vi "_FPGA Set Parameters.vi"(4 "HV Only (F)":bool, 5 "Source Standby (F)":bool, 6 "ExhaustGas (on)":bool=TRUE, 7 "CurGas (on)":bool=TRUE, 8 "error in":errorcluster, 9 "Set Zero (on)":bool=TRUE, 10 "HSID Temp (on)":bool=TRUE) -> (0 "error out":errorcluster)   [LabVIEW 2012]
uses:
  Type/_RT Active Ch.ctl
  Type/_RT Parameter.ctl
  Type/_RT Expt.ctl
  Type/_Run Mode.ctl
  Type/_RT Mass Range.ctl
  Type/_RT Res Type.ctl
  Type/_FPGA Indicator.ctl
  _RT Global.vi
  <vilib>/Utility/error.llb/Error Cluster From Error Code.vi
  <vilib>/rvi/errors/niLvFpgaAdjustHostInterfaceError.vi
  <vilib>/rvi/interface/nirviReadWriteControl/nirviReadWriteControl.xnode
  FPGA Bitfiles/FPGA9606.lvbitx
  NiFpgaLv.dll
panel:
  out "Array":T1[](array[typedef])
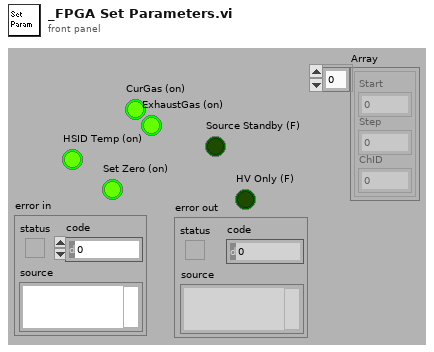
[diagram p1: front panel]
types:
  T1 = typedef "_RT Active Ch.ctl" = cluster{"Start":i32, "Step":i32, "ChID":i32}
  T2 = typedef "_RT Expt.ctl" = cluster{"StartT(mS)":i32, "#Cycles":i32, "Scan Type":T3, "PauseT(uS)":i32, "Polarity":u8, "DelayT(mS)":i32, "Active Ch":T1[], "Mass Range":T4[]}
  T3 = typedef "_Run Mode.ctl" = enum16{"MRM (Q1/Q2)", "Q1 Scan", "Q1 SRM", "Q2 Scan", "Q2 SRM", "Product Scan", "Precursor Scan", "Neutral Loss", "Neutral Gain"}
  T4 = typedef "_RT Mass Range.ctl" = cluster{"Steps":i32, "Dwell(uS)":i32, "Resolution Type":T5, "Ramping Ch":T1[]}
  T5 = typedef "_RT Res Type.ctl" = u16
  T6 = typedef "_RT Parameter.ctl" = cluster{"RunMode":i32, "Initial Ch":T1[], "Sync":u8, "Expt":T2[], "EqTime(mS)":i32}
  T7 = typedef "_RT Instrument 2.ctl" = cluster{"Table":T8[], "Instrument":string[]}
  T8 = typedef "_RT Configuration 2.ctl" = cluster{"Name":string, "Ch#":u8, "Min":dbl, "Max":dbl, "Def+":dbl, "Def-":dbl, "Offset":dbl, "Slope":dbl, "Type":u8, "Description":string, "SettleT":dbl}
  T9 = typedef "Semaphore RefNum" = refnum<k1>
  T10 = typedef "_FPGA Indicator.ctl" = enum16{"Done", "Ready", "Count Available", "SendSerial", "LED State"}
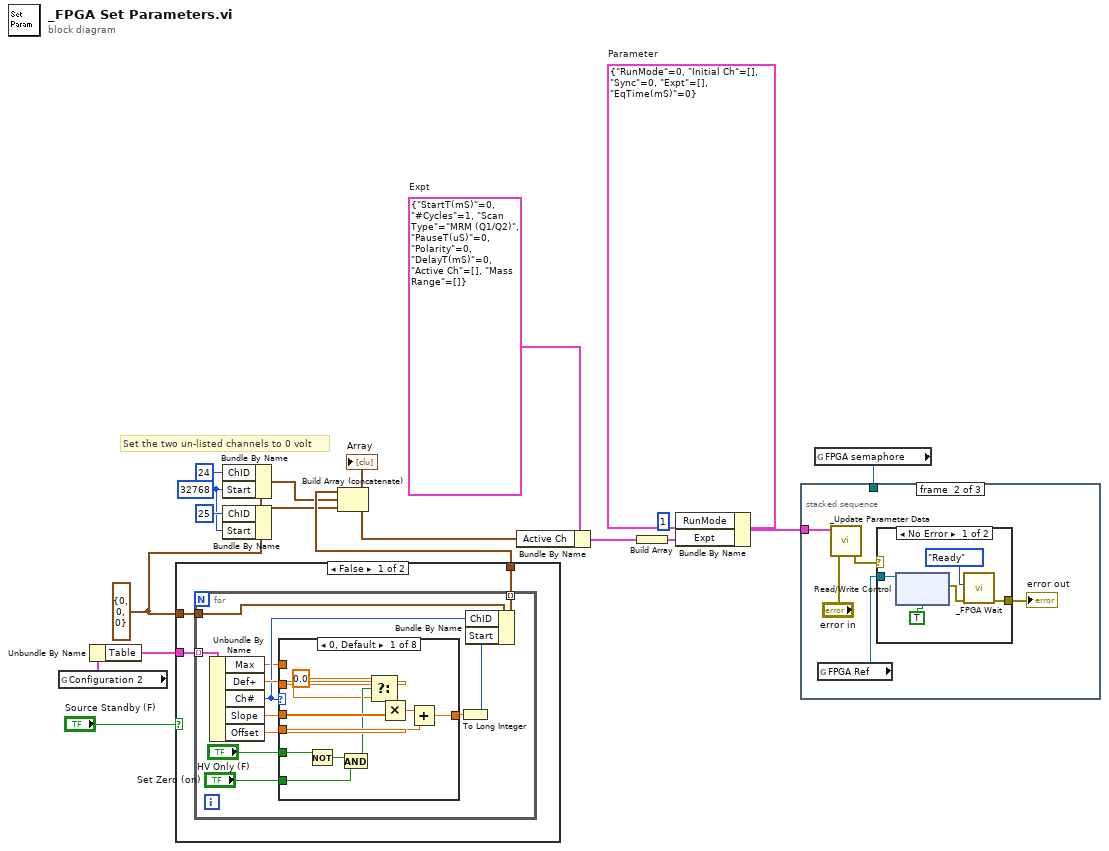
[diagram p0: block diagram]
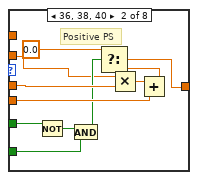
[diagram p2: hidden frame]
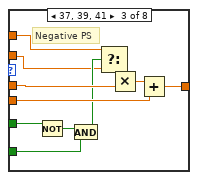
[diagram p3: hidden frame]
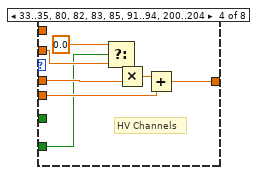
[diagram p4: hidden frame]
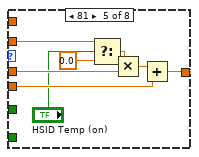
[diagram p5: hidden frame]
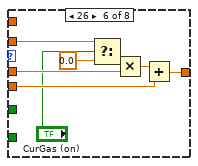
[diagram p6: hidden frame]
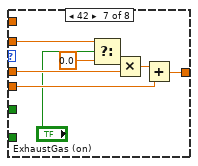
[diagram p7: hidden frame]
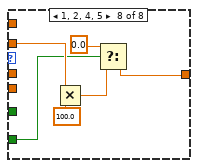
[diagram p8: hidden frame]
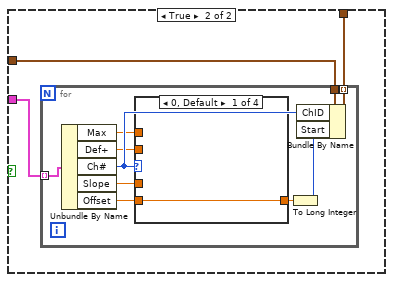
[diagram p9: hidden frame]
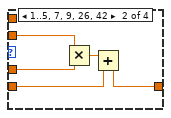
[diagram p10: hidden frame]
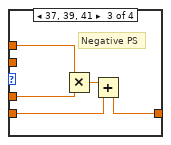
[diagram p11: hidden frame]
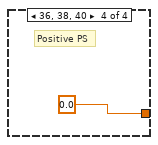
[diagram p12: hidden frame]
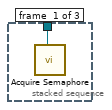
[diagram p13: hidden frame]
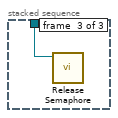
[diagram p15: hidden frame]
diagram:
  w5 = 32768 ("Start")
  w8 = T1 {"Start"=0, "Step"=0, "ChID"=0} ("Active Channel")
  w16 = T2 {"StartT(mS)"=0, "#Cycles"=1, "Scan Type"=enum."MRM (Q1/Q2)", "PauseT(uS)"=0, "Polarity"=0, "DelayT(mS)"=0, "Active Ch"=[], "Mass Range"=[]}  # Expt
  w15 = T6 {"RunMode"=0, "Initial Ch"=[], "Sync"=0, "Expt"=[], "EqTime(mS)"=0}  # Parameter
  # "Set the two un-listed channels to 0 volt"
  n1 = global read "_RT Global.vi" "Configuration 2"() -> (w11:T7)
  n2 = Unbundle By Name(w11) -> ("Table"=w17:T8[])
  n3 = case shown="False" "Source Standby (F)" {
    tunnel: [w21 w105] -> w4
    tunnel: w17 -> [w20 w106]
    tunnel: w8 -> [w19 w107]
    frame False {
      n4 = for {
        tunnel: w20 -> [w33] mode=indexing
        tunnel: [w32] -> w21 mode=indexing
        tunnel: w19 -> [w24]
        n5 = Unbundle By Name(w33) -> ("Max"=w22:dbl, "Def+"=w31:dbl, "Ch#"=w26:u8, "Slope"=w30:dbl, "Offset"=w29:dbl)
        n6 = case shown="0, Default" w26 {
          tunnel: w31 -> [w36 w47 w57 w70 w77 w84 w92 w103]
          tunnel: w30 -> [w44 w55 w66 w74 w82 w90 w98 _]
          tunnel: w29 -> [w43 w54 w65 w73 w81 w89 w97 _]
          tunnel: [w34 w45 w62 w68 w76 w85 w93 w99] -> w28
          tunnel: "Set Zero (on)" -> [w39 w50 w60 w67 _ _ _ w102]
          tunnel: "HV Only (F)" -> [w37 w48 w58 _ _ _ _ _]
          tunnel: w22 -> [_ _ w56 _ _ _ _ _]
          frame 0, Default {
            n7 = Not(x=w37) -> (.not. x?=w40:bool)
            n8 = And(x=w40, y=w39) -> (x .and. y?=w38:bool)
            n9 = Select(t=0.0 ("f"), s=w38, f=w36) -> (s? t:f=w35:dbl)
            n10 = Multiply(x=w35, y=w44) -> (x*y=w42:dbl)
            n11 = Add(x=w42, y=w43) -> (x+y=w34:dbl)
          }
          frame 36, 38, 40 {
            # "Positive PS"
            n12 = Not(x=w48) -> (.not. x?=w51:bool)
            n13 = And(x=w51, y=w50) -> (x .and. y?=w49:bool)
            n14 = Multiply(x=w47, y=w55) -> (x*y=w53:dbl)
            n15 = Add(x=w53, y=w54) -> (x+y=w46:dbl)
            n16 = Select(t=0.0 ("f"), s=w49, f=w46) -> (s? t:f=w45:dbl)
          }
          frame 37, 39, 41 {
            # "Negative PS"
            n17 = Not(x=w58) -> (.not. x?=w61:bool)
            n18 = And(x=w61, y=w60) -> (x .and. y?=w59:bool)
            n19 = Select(t=w56, s=w59, f=w57) -> (s? t:f=w63:dbl)
            n20 = Multiply(x=w63, y=w66) -> (x*y=w64:dbl)
            n21 = Add(x=w64, y=w65) -> (x+y=w62:dbl)
          }
          frame 33..35, 80, 82, 83, 85, 91..94, 200..204 {
            # "HV Channels"
            n22 = Select(t=0.0 ("f"), s=w67, f=w70) -> (s? t:f=w69:dbl)
            n23 = Multiply(x=w69, y=w74) -> (x*y=w72:dbl)
            n24 = Add(x=w72, y=w73) -> (x+y=w68:dbl)
          }
          frame 81 {
            n25 = Select(t=w77, s="HSID Temp (on)", f=0.0) -> (s? t:f=w75:dbl)
            n26 = Multiply(x=w75, y=w82) -> (x*y=w80:dbl)
            n27 = Add(x=w80, y=w81) -> (x+y=w76:dbl)
          }
          frame 26 {
            n28 = Select(t=w84, s="CurGas (on)", f=0.0) -> (s? t:f=w83:dbl)
            n29 = Multiply(x=w83, y=w90) -> (x*y=w88:dbl)
            n30 = Add(x=w88, y=w89) -> (x+y=w85:dbl)
          }
          frame 42 {
            n31 = Select(t=w92, s="ExhaustGas (on)", f=0.0) -> (s? t:f=w91:dbl)
            n32 = Multiply(x=w91, y=w98) -> (x*y=w96:dbl)
            n33 = Add(x=w96, y=w97) -> (x+y=w93:dbl)
          }
          frame 1, 2, 4, 5 {
            n34 = Multiply(x=w103, y=100.0) -> (x*y=w100:dbl)
            n35 = Select(t=0.0 ("y"), s=w102, f=w100) -> (s? t:f=w99:dbl)
          }
        }
        n36 = To Long Integer(number=w28) -> (32bit integer=w27:i32)
        n37 = Bundle By Name(cluster=w24, "ChID"=w26, "Start"=w27) -> (w32:T1)
      }
    }
    frame True {
      n38 = for {
        tunnel: w107 -> [w111]
        tunnel: w106 -> [w110] mode=indexing
        tunnel: [w109] -> w105 mode=indexing
        n39 = Unbundle By Name(w110) -> ("Max"=w108:dbl, "Def+"=w113:dbl, "Ch#"=w114:u8, "Slope"=w112:dbl, "Offset"=w117:dbl)
        n40 = case shown="0, Default" w114 {
          tunnel: [w118 w119 w125 0.0 ("Offset")] -> w116
          tunnel: w117 -> [w118 w120 w126 _]
          tunnel: w113 -> [_ w122 _ _]
          tunnel: w112 -> [_ w121 w127 _]
          tunnel: w108 -> [_ _ w124 _]
          frame 0, Default {
          }
          frame 1..5, 7, 9, 26, 42 {
            n41 = Multiply(x=w122, y=w121) -> (x*y=w123:dbl)
            n42 = Add(x=w123, y=w120) -> (x+y=w119:dbl)
          }
          frame 37, 39, 41 {
            # "Negative PS"
            n43 = Multiply(x=w124, y=w127) -> (x*y=w128:dbl)
            n44 = Add(x=w128, y=w126) -> (x+y=w125:dbl)
          }
          frame 36, 38, 40 {
            # "Positive PS"
          }
        }
        n45 = To Long Integer(number=w116) -> (32bit integer=w115:i32)
        n46 = Bundle By Name(cluster=w111, "ChID"=w114, "Start"=w115) -> (w109:T1)
      }
    }
  }
  n47 = Bundle By Name(cluster=w8, "ChID"=24, "Start"=w5) -> (w3:T1)
  n48 = Bundle By Name(cluster=w8, "ChID"=25, "Start"=w5) -> (w2:T1)
  n49 = Build Array (concatenate)(w4, w3, w2) -> (w1:T1[])
  "Array" <- w1
  n50 = Bundle By Name(cluster=w16, "Active Ch"=w1) -> (w13:T2)
  n51 = Build Array(w13) -> (w14:T2[])
  n52 = Bundle By Name(cluster=w15, "RunMode"=1, "Expt"=w14) -> (w18:T6)
  n53 = global read "_RT Global.vi" "FPGA semaphore"() -> (w10:T9)
  n54 = stacked-sequence {
    tunnel: w18 -> [_ w134 _]
    tunnel: w10 -> [w130 _ w142]
    frame #0 {
      n55 = call <vilib>:"Acquire Semaphore.vi"("semaphore"=w130) -> ()  [unwired: 2 in, 5 out]
    }
    frame #1 {
      n56 = global read "_RT Global.vi" "FPGA Ref"() -> (w131:refnum<k20>)
      n57 = call "_Update Parameter Data.vi"("error in"="error in", "Parameter"=w134) -> ("error out"=w135:errorcluster)  [unwired: 1 in, 4 out]
      n58 = case shown="No Error" w135 {
        selector: w135 -> [_ w141]
        tunnel: w131 -> [w140 _]
        tunnel: [w137 w141] -> w133
        frame No Error {
          n59 = xnode "Read/Write Control"("FPGA VI Reference In"=w140, "Start"=TRUE) -> ("error out"=w136:errorcluster)  [unwired: 1 in, 1 out]
          n60 = call "_FPGA Wait.vi"("error in"=w136, "Indicator"=_FPGA_Indicator."Ready") -> ("error out"=w137:errorcluster)  [unwired: 3 in, 2 out]
        }
        frame Error {
        }
      }
      "error out" <- w133
    }
    frame #2 {
      n61 = call <vilib>:"Release Semaphore.vi"("semaphore"=w142) -> ()  [unwired: 1 in, 6 out]
    }
  }
